vi "TAT_ IO Status.vi"(8 "error in (no error)":errorcluster) -> (0 "error out":errorcluster)   [LabVIEW 2017]
uses:
  <vilib>/NI/Modbus Library/API/Wrapper/Create TCP Master.vi
  <vilib>/NI/Modbus Library/API/Master/Modbus Master.lvclass
  <vilib>/NI/Modbus Library/API/Wrapper/API Main.lvlib
panel:
  in  "Tab Control":enum32{"INPUTS", "OUTPUTS"}(tab)
  out "Stud Present-03":bool
  out "Child Part-02":bool
  out "Child Part-03":bool
  out "Child Part-04":bool
  out "Child Part-05":bool
  out "Child Part-06":bool
  out "Child Part-07":bool
  out "Child Part-08":bool
  out "Stud Present-01":bool
  out "Stud Present-02":bool
  out "Child Part-01":bool
  out "St-02 Bin-01":bool
  out "St-02 Bin-02":bool
  out "St-02 Bin-03":bool
  out "St-02 Bin-04":bool
  out "St-02 Bin-05":bool
  out "St-02 Bin-06":bool
  out "Cycle Start-1":bool
  out "Cycle Start-2":bool
  out "Reset":bool
  out "Emergency Stop":bool
  out "Fixture Present-01":bool
  out "Fixture Present-02":bool
  out "Fixture Present-03":bool
  out "Stoke Mid Pos-V1":bool
  out "Stroke Low Pos-V1":bool
  out "Stroke Hi Pos-V1":bool
  out "Stroke Mid Pos-V2":bool
  out "Stroke Low Pos-V2":bool
  out "Stroke Hi Pos-V2":bool
  in  "Red Tower Lamp":bool
  in  "Buzzer Tower Lamp":bool
  in  "Yellow Tower Lamp":bool
  in  "Green Tower Lamp":bool
  in  "Ram Cyl Up Coil-01":bool
  in  "Ram Cyl Dn Coil-01":bool
  in  "Ram Cyl Up Coil-02":bool
  in  "Ram Cyl Dn Coil-02":bool
  in  "Part Clamp Cyl":bool
  in  "Dot Punch Cyl":bool
  in  "St-02 Bin-01":bool
  in  "St-02 Bin-02":bool
  in  "St-02 Bin-03":bool
  in  "St-02 Bin-04":bool
  in  "St-02 Bin-05":bool
  in  "St-02 Bin-06":bool
  in  "stop":bool
  # "STATION IO STATUS"
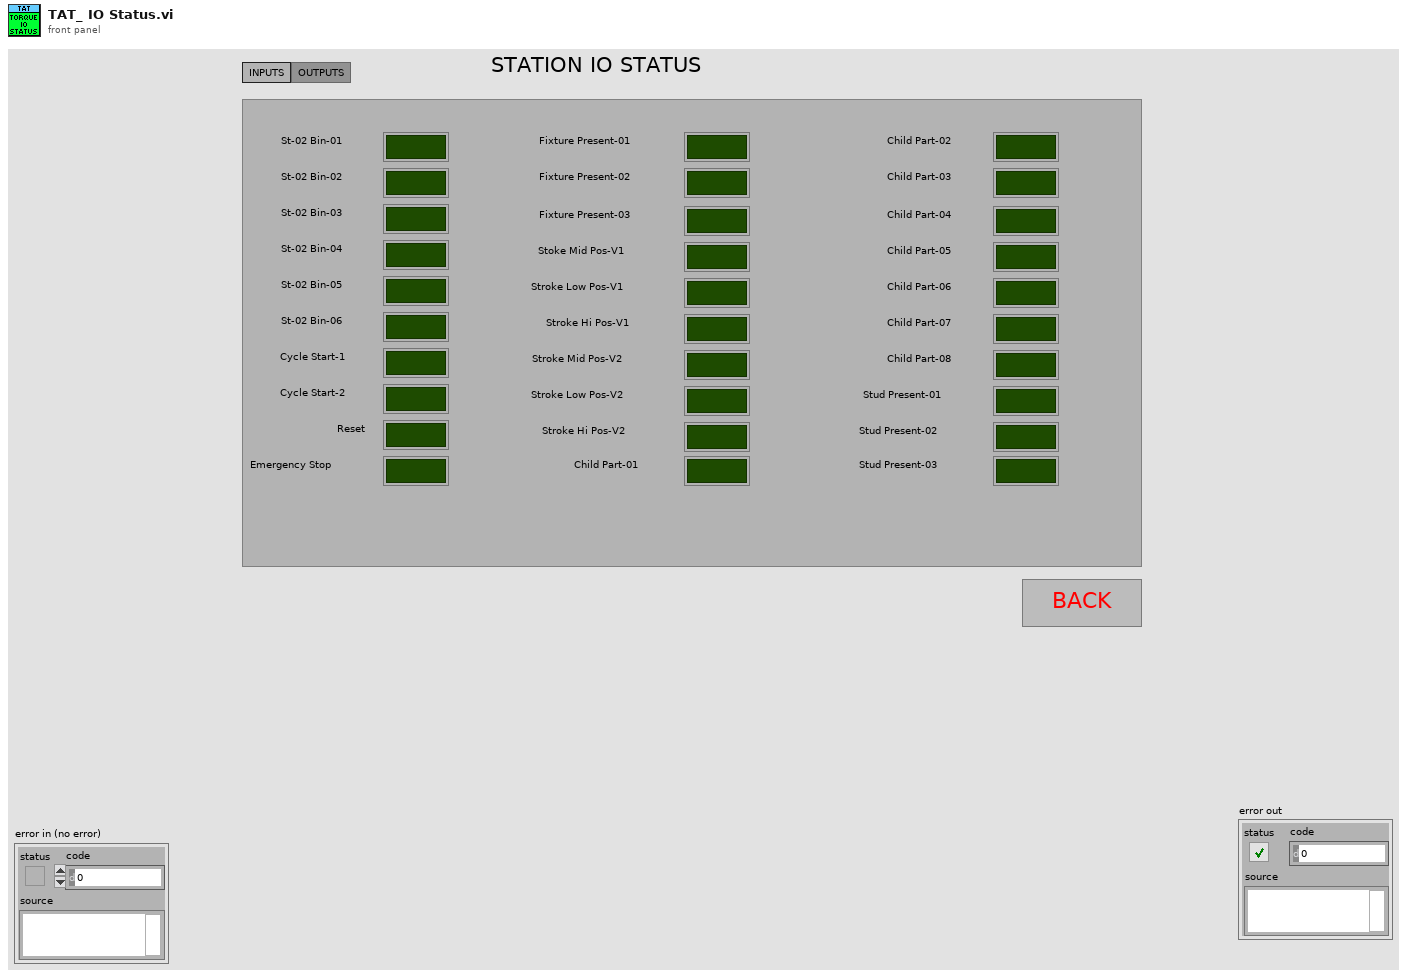
[diagram p1: front panel]
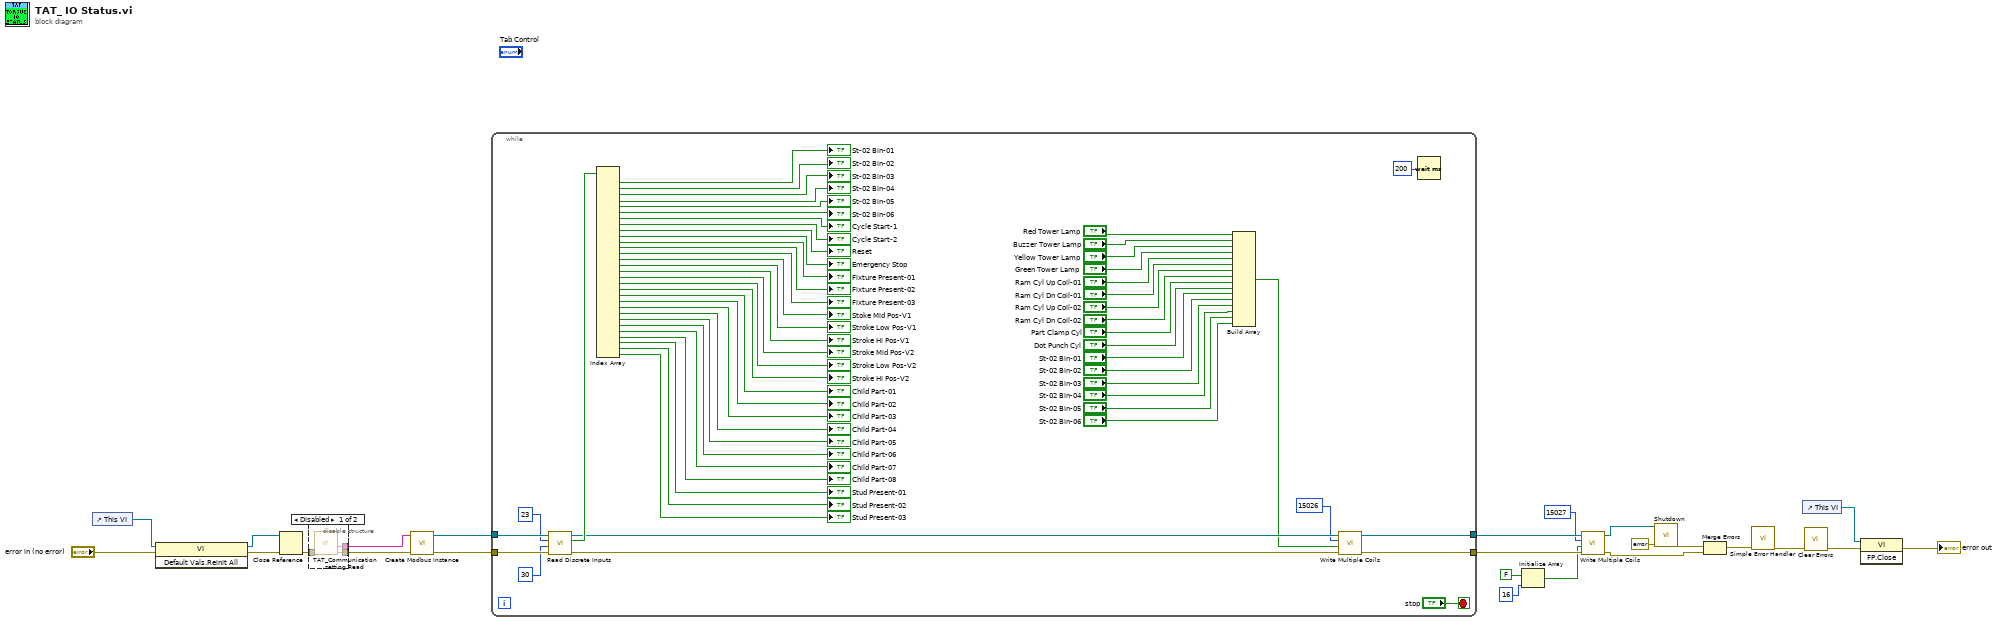
[diagram p0: block diagram]
diagram:
  n1 = control-ref of="This VI"() -> (w5:refnum<vi>)
  n2 = invoke class="VI" method="Default Vals.Reinit All"(reference=w5, error in="error in (no error)") -> (reference out=w3:refnum<vi>, error out=w2:errorcluster)  [unwired: 1 in, 1 out]
  n3 = Close Reference(reference=w3, error in (no error)=w2) -> (error out=w1:errorcluster)
  n4 = disable-structure shown="Disabled" {
    disable-tunnel: [w27 _] -> w24
    disable-tunnel: [w26 _] -> w23
    disable-tunnel: w1 -> [w25 _]
    frame Disabled {
      n5 = call "TAT_Communication setting Read.vi"("error in (no error)"=w25) -> ("error out"=w27:errorcluster, "PLC IP"=w26:string)  [unwired: 3 in, 6 out]
    }
    frame Enabled {
    }
  }
  n6 = call-poly <vilib>:"Create Modbus Instance.vi"("error in"=w24, "address"=w23) -> ("error out"=w22:errorcluster, "TCP master instance"=w21:refnum<class "Modbus Master.lvclass">)  [unwired: 8 in]
  n7 = while {
    tunnel: w22 -> [w85]
    tunnel: w21 -> [w84]
    tunnel: [w45] -> w11
    tunnel: [w44] -> w13
    stop <- "stop" stop-if-true
    n8 = call-dynamic "Read Discrete Inputs.vi"("error in"=w85, "number of inputs"=u16 30, "starting address"=u16 23, "Modbus master in"=w84) -> ("error out"=w59:errorcluster, "discrete inputs"=w81:bool[], "Modbus master out"=w60:refnum<class "Modbus Master.lvclass">)  [unwired: 5 in]
    n9 = Index Array(array=w81) -> (element #1=→"St-02 Bin-01":bool, element #2=→"St-02 Bin-02":bool, element #3=→"St-02 Bin-03":bool, element #4=→"St-02 Bin-04":bool, element #5=→"St-02 Bin-05":bool, element #6=→"St-02 Bin-06":bool, element #7=→"Cycle Start-1":bool, element #8=→"Cycle Start-2":bool, element #9=→"Reset":bool, element #10=→"Emergency Stop":bool, element #11=→"Fixture Present-01":bool, element #12=→"Fixture Present-02":bool, element #13=→"Fixture Present-03":bool, element #14=→"Stoke Mid Pos-V1":bool, element #15=→"Stroke Low Pos-V1":bool, element #16=→"Stroke Hi Pos-V1":bool, element #17=→"Stroke Mid Pos-V2":bool, element #18=→"Stroke Low Pos-V2":bool, element #19=→"Stroke Hi Pos-V2":bool, element #20=→"Child Part-01":bool, element #21=→"Child Part-02":bool, element #22=→"Child Part-03":bool, element #23=→"Child Part-04":bool, element #24=→"Child Part-05":bool, element #25=→"Child Part-06":bool, element #26=→"Child Part-07":bool, element #27=→"Child Part-08":bool, element #28=→"Stud Present-01":bool, element #29=→"Stud Present-02":bool, element #30=→"Stud Present-03":bool)  [unwired: 30 in]
    n10 = Build Array("Red Tower Lamp", "Buzzer Tower Lamp", "Yellow Tower Lamp", "Green Tower Lamp", "Ram Cyl Up Coil-01", "Ram Cyl Dn Coil-01", "Ram Cyl Up Coil-02", "Ram Cyl Dn Coil-02", "Part Clamp Cyl", "Dot Punch Cyl", "St-02 Bin-01", "St-02 Bin-02", "St-02 Bin-03", "St-02 Bin-04", "St-02 Bin-05", "St-02 Bin-06") -> (w46:bool[])
    n11 = call-dynamic "Write Multiple Coils.vi"("error in"=w59, "coils to write"=w46, "starting address"=u16 15026, "Modbus master in"=w60) -> ("error out"=w45:errorcluster, "Modbus master out"=w44:refnum<class "Modbus Master.lvclass">)  [unwired: 6 in]
    n12 = Wait (ms)(milliseconds to wait=u32 200) -> ()  [unwired: 1 out]
  }
  n13 = Initialize Array(FALSE, 16 ("dimension size")) -> (w6:bool[])
  n14 = call-dynamic "Write Multiple Coils.vi"("error in"=w11, "coils to write"=w6, "starting address"=u16 15027, "Modbus master in"=w13) -> ("error out"=w10:errorcluster, "Modbus master out"=w12:refnum<class "Modbus Master.lvclass">)  [unwired: 6 in]
  n15 = call-dynamic "Shutdown.vi"("error in"=errorcluster {"status"=FALSE, "code"=0, "source"=""}, "Modbus master in"=w12) -> ("error out"=w19:errorcluster)  [unwired: 9 in]
  n16 = Merge Errors(w19, w10) -> (w18:errorcluster)
  n17 = call <vilib>:"Simple Error Handler.vi"("error in (no error)"=w18) -> ("error out"=w17:errorcluster)  [unwired: 4 in, 4 out]
  n18 = control-ref of="This VI"() -> (w15:refnum<vi>)
  n19 = call <vilib>:"Clear Errors.vi"("error in (no error)"=w17) -> ("error out"=w16:errorcluster)  [unwired: 5 in, 1 out]
  n20 = invoke class="VI" method="FP.Close"(reference=w15, error in=w16) -> (error out=→"error out":errorcluster)  [unwired: 1 in, 2 out]
